vi "Send Arm Acquisition Engine.vi"(8 "error in":errorcluster, 11 "FPGA VI Reference In":refnum<k20>) -> (0 "error out":errorcluster, 3 "FPGA VI Reference Out":refnum<k20>)   [LabVIEW 2012]
uses:
  <vilib>/Utility/error.llb/Error Cluster From Error Code.vi
  <vilib>/rvi/errors/niLvFpgaAdjustHostInterfaceError.vi
  <vilib>/rvi/interface/nirviReadWriteControl/nirviReadWriteControl.xnode
  NiFpgaLv.dll
  <vilib>/rvi/interface/Simulation/niFpgaSimulationCallBeginRW.vi
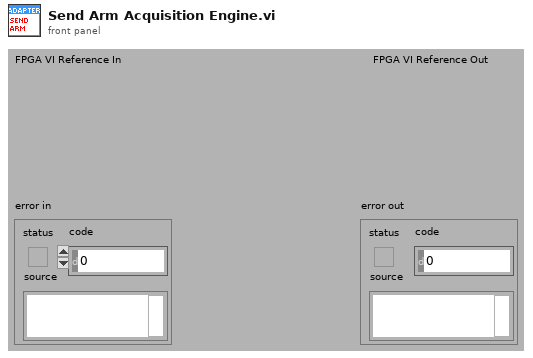
[diagram p1: front panel]
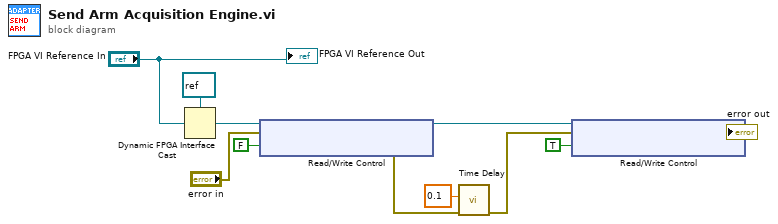
[diagram p0: block diagram]
diagram:
  n1 = Dynamic FPGA Interface Cast(Session In=refnum<k20> refnum ("Type"), Type="FPGA VI Reference In") -> (Session Out=w5:refnum<k20>)
  n2 = xnode "Read/Write Control"("FPGA VI Reference In"=w5, "error in"="error in", "Arm Acquisition Engine"=FALSE ("Reset?")) -> ("FPGA VI Reference Out"=w8:refnum<k20>, "error out"=w3:errorcluster)
  n3 = call "Time Delay"("error in (no error)"=w3, "Delay Time (s)"=0.1) -> ("error out"=w2:errorcluster)  [unwired: 9 in]
  n4 = xnode "Read/Write Control"("FPGA VI Reference In"=w8, "error in"=w2, "Arm Acquisition Engine"=TRUE ("Reset?")) -> ("error out"=→"error out":errorcluster)  [unwired: 1 out]
  "FPGA VI Reference Out" <- "FPGA VI Reference In"
